vi "Rotate Map.vi"(8 "error in (no error)":errorcluster, 10 "Rotation Angle":dbl, 11 "Map Model in":refnum<class "Map Model.lvclass">) -> (0 "error out":errorcluster, 3 "Map Model out":refnum<class "Map Model.lvclass">)   [LabVIEW 2020, in "Map Model.lvlib" / "Map Model.lvclass"]
uses:
  Map Model.lvclass
  Map Model.lvclass/Map Model.ctl
  Tools/Tool/Tool.lvclass/Tool.ctl
  Tools/Tool/Tool.lvclass
  Stack/Stack.lvclass
panel:
  # "NOTICE -- YOU MUST LEAVE THIS NOTICE IN PLACE.\n\nCopyright (c) 2017, LIANG LIU Shawn.Liu.cn@gmail.com\nAll rights reserved.\n\nRedistribution and use in source and binary forms, with or without modification, are permitted provided that the following conditions are met:\n-Redistributions of source code must retain the above copyright notice, this list of conditions and the following disclaimer.\n-Redistributions in binary form must reproduce the above copyright notice, this list of conditions and the following disclaimer in the documentation and/or other materials provided with the distribution.\n-Neither the name of the eLp nor the names of its contributors may be used to endorse or promote products derived from this software without specific prior written permission.\n\nTHIS SOFTWARE IS PROVIDED BY THE COPYRIGHT HOLDERS AND CONTRIBUTORS \"AS IS\" AND ANY EXPRESS OR IMPLIED WARRANTIES, INCLUDING, BUT NOT LIMITED TO, THE IMPLIED WARRANTIES OF MERCHANTABILITY AND FITNESS FOR A PARTICULAR PURPOSE ARE DISCLAIMED. IN NO EVENT SHALL THE COPYRIGHT HOLDER OR CONTRIBUTORS BE LIABLE FOR ANY DIRECT, INDIRECT, INCIDENTAL, SPECIAL, EXEMPLARY, OR CONSEQUENTIAL DAMAGES (INCLUDING, BUT NOT LIMITED TO, PROCUREMENT OF SUBSTITUTE GOODS OR SERVICES; LOSS OF USE, DATA, OR PROFITS; OR BUSINESS INTERRUPTION) HOWEVER CAUSED AND ON ANY THEORY OF LIABILITY, WHETHER IN CONTRACT, STRICT LIABILITY, OR TORT (INCLUDING NEGLIGENCE OR OTHERWISE) ARISING IN ANY WAY OUT OF THE USE OF THIS SOFTWARE, EVEN IF ADVISED OF THE POSSIBILITY OF SUCH DAMAGE."
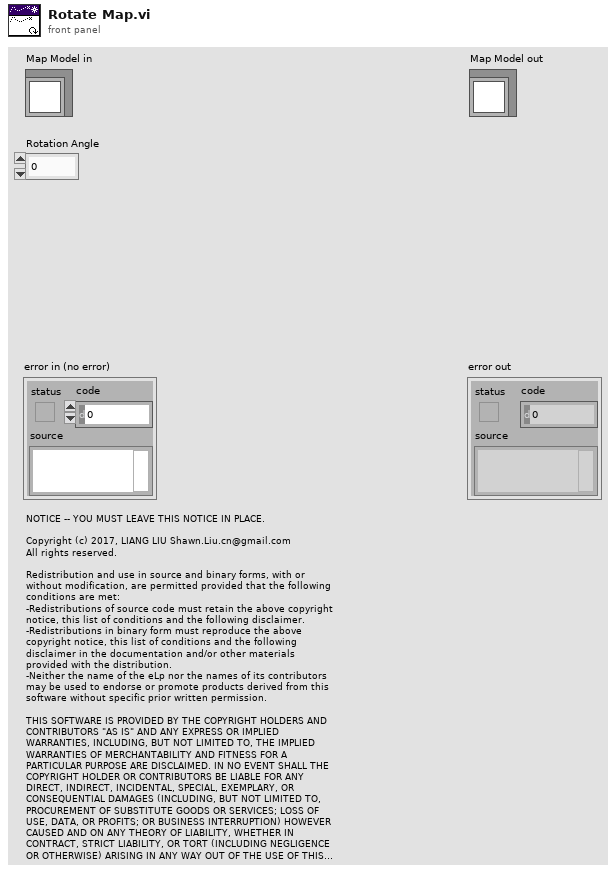
[diagram p1: front panel]
types:
  T1 = enum8{"Enabled", "Disabled", "Disabled and Grayed Out"}
  T2 = typedef "LVPoint32TypeDef.ctl" = cluster{"Horizontal":i32, "Vertical":i32}
  T3 = typedef "LVPointTypeDef.ctl" = cluster{"Horizontal":i16, "Vertical":i16}
  T4 = cluster{"Occupied Color":cluster{"Value":u8, "Color":u32}, "Free Color":cluster{"Value":u8, "Color":u32}, "Unknown Color":cluster{"Value":u8, "Color":u32}}
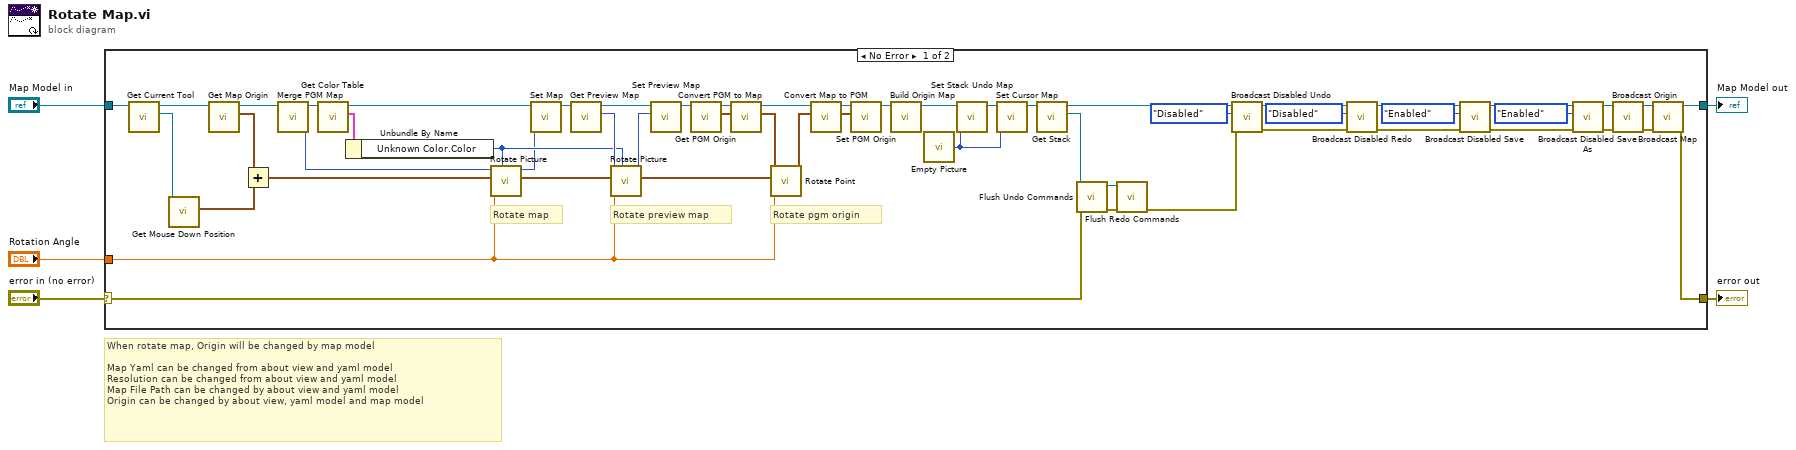
[diagram p0: block diagram]
diagram:
  # "When rotate map, Origin will be changed by map model\n\nMap Yaml can be changed from about view and yaml model\nResolution can be changed from about view and yaml model\nMap File Path can be changed by about view and yaml model\nOrigin can be changed by about view, yaml model and map model"
  n1 = case shown="No Error" "error in (no error)" {
    selector: "error in (no error)" -> [w54 w60]
    tunnel: "Map Model in" -> [w58 w59]
    tunnel: [w57 w60] -> w4
    tunnel: [w56 w59] -> w3
    tunnel: "Rotation Angle" -> [w55 _]
    frame No Error {
      # "Rotate pgm origin"
      # "Rotate preview map"
      # "Rotate map"
      n2 = call "Get Current Tool.vi"("Map Model in"=w58) -> ("Current Tool"=w51:refnum<class "Tool.lvclass">, "Map Model out"=w52:refnum<class "Map Model.lvclass">)  [unwired: 9 in]
      n3 = call "Get Mouse Down Position.vi"("Tool in"=w51) -> ("Mouse Down Position"=w46:T2)  [unwired: 9 in, 1 out]
      n4 = call "Get Map Origin.vi"("Map Model in"=w52) -> ("Map Origin"=w47:T3, "Map Model out"=w48:refnum<class "Map Model.lvclass">)  [unwired: 9 in]
      n5 = Add(x=w47, y=w46) -> (x+y=w28:T2)
      n6 = call "Merge PGM Map.vi"("Map Model in"=w48) -> ("Map"=w45:picture, "Map Model out"=w53:refnum<class "Map Model.lvclass">)  [unwired: 7 in, 2 out]
      n7 = call "Get Color Table.vi"("Map Model in"=w53) -> ("Color Table"=w49:T4, "Map Model out"=w50:refnum<class "Map Model.lvclass">)  [unwired: 9 in]
      n8 = Unbundle By Name(w49) -> ("Unknown Color.Color"=w31:u32)
      n9 = call "Rotate Picture.vi"("Unknown Color (black)"=w31, "Rotation Angle (degree)"=w55, "Center"=w28, "Picture in"=w45) -> ("Picture out"=w8:picture)  [unwired: 7 in]
      n10 = call "Set Map.vi"("Map"=w8, "Map Model in"=w50) -> ("Map Model out"=w7:refnum<class "Map Model.lvclass">)  [unwired: 9 in]
      n11 = call "Get Preview Map.vi"("Map Model in"=w7) -> ("Preview Map"=w32:picture, "Map Model out"=w34:refnum<class "Map Model.lvclass">)  [unwired: 9 in]
      n12 = call "Rotate Picture.vi"("Unknown Color (black)"=w31, "Rotation Angle (degree)"=w55, "Center"=w28, "Picture in"=w32) -> ("Picture out"=w30:picture)  [unwired: 7 in]
      n13 = call "Set Preview Map.vi"("Preview Map"=w30, "Map Model in"=w34) -> ("Map Model out"=w33:refnum<class "Map Model.lvclass">)  [unwired: 9 in]
      n14 = call "Get PGM Origin.vi"("Map Model in"=w33) -> ("PGM Origin"=w12:cluster{"Horizontal":dbl, "Vertical":dbl}, "Map Model out"=w13:refnum<class "Map Model.lvclass">)  [unwired: 9 in]
      n15 = call "Convert PGM to Map.vi"("Position on PGM"=w12, "Map Model in"=w13) -> ("Position on Map"=w27:T3, "Map Model out"=w29:refnum<class "Map Model.lvclass">)  [unwired: 8 in]
      n16 = call "Rotate Point.vi"("Rotation Angle (degree)"=w55, "Center"=w28, "Point in"=w27) -> ("Point out"=w10:cluster{"X":i32, "Y":i32})  [unwired: 8 in]
      n17 = call "Convert Map to PGM.vi"("Position on Map"=w10, "Map Model in"=w29) -> ("Position on PGM"=w9:T3, "Map Model out"=w26:refnum<class "Map Model.lvclass">)  [unwired: 8 in]
      n18 = call "Set PGM Origin.vi"("PGM Origin"=w9, "Map Model in"=w26) -> ("Map Model out"=w11:refnum<class "Map Model.lvclass">)  [unwired: 9 in]
      n19 = call "Build Origin Map.vi"("Map Model in"=w11) -> ("Map Model out"=w6:refnum<class "Map Model.lvclass">)  [unwired: 9 in, 1 out]
      n20 = call "Empty Picture"() -> ("empty picture"=w15:picture)
      n21 = call "Set Stack Undo Map.vi"("Stack Undo Map"=w15, "Map Model in"=w6) -> ("Map Model out"=w44:refnum<class "Map Model.lvclass">)  [unwired: 9 in]
      n22 = call "Set Cursor Map.vi"("Cursor Map"=w15, "Map Model in"=w44) -> ("Map Model out"=w14:refnum<class "Map Model.lvclass">)  [unwired: 9 in]
      n23 = call "Get Stack.vi"("Map Model in"=w14) -> ("Stack"=w35:refnum<class "Stack.lvclass">, "Map Model out"=w38:refnum<class "Map Model.lvclass">)  [unwired: 9 in]
      n24 = call "Flush Undo Commands.vi"("error in (no error)"=w54, "Stack in"=w35) -> ("error out"=w43:errorcluster, "Stack out"=w42:refnum<class "Stack.lvclass">)  [unwired: 8 in]
      n25 = call "Flush Redo Commands.vi"("error in (no error)"=w43, "Stack in"=w42) -> ("error out"=w36:errorcluster)  [unwired: 8 in, 1 out]
      n26 = call "Broadcast Disabled Undo.vi"("error in (no error)"=w36, "Disabled Undo"=T1."Disabled", "Map Model in"=w38) -> ("error out"=w37:errorcluster, "Map Model out"=w41:refnum<class "Map Model.lvclass">)  [unwired: 7 in]
      n27 = call "Broadcast Disabled Redo.vi"("error in (no error)"=w37, "Disabled Redo"=T1."Disabled", "Map Model in"=w41) -> ("error out"=w24:errorcluster, "Map Model out"=w18:refnum<class "Map Model.lvclass">)  [unwired: 7 in]
      n28 = call "Broadcast Disabled Save.vi"("error in (no error)"=w24, "Disabled Save"=T1."Enabled", "Map Model in"=w18) -> ("error out"=w23:errorcluster, "Map Model out"=w25:refnum<class "Map Model.lvclass">)  [unwired: 7 in]
      n29 = call "Broadcast Disabled Save As.vi"("error in (no error)"=w23, "Disabled Save As"=T1."Enabled", "Map Model in"=w25) -> ("error out"=w21:errorcluster, "Map Model out"=w22:refnum<class "Map Model.lvclass">)  [unwired: 7 in]
      n30 = call "Broadcast Origin.vi"("error in (no error)"=w21, "Map Model in"=w22) -> ("error out"=w19:errorcluster, "Map Model out"=w20:refnum<class "Map Model.lvclass">)  [unwired: 8 in]
      n31 = call "Broadcast Map.vi"("error in (no error)"=w19, "Map Model in"=w20) -> ("error out"=w57:errorcluster, "Map Model out"=w56:refnum<class "Map Model.lvclass">)  [unwired: 8 in]
    }
    frame Error {
    }
  }
  "error out" <- w4
  "Map Model out" <- w3
